vi "例4-7.vi"() -> ()   [LabVIEW 2019]
panel:
  out "所用时间9ms)":dbl
  out "执行次数":dbl
  in  "给定数据":dbl=50.0
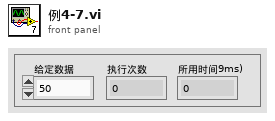
[diagram p1: front panel]
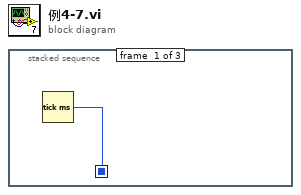
[diagram p0: block diagram]
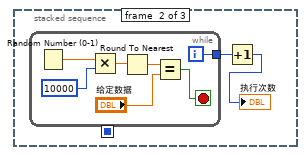
[diagram p2: hidden frame]
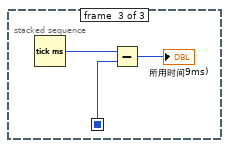
[diagram p3: hidden frame]
diagram:
  n1 = stacked-sequence {
    seq-local: [w1 _ _] -> [_ _ w12]
    frame #0 {
      n2 = Tick Count (ms)() -> (millisecond timer value=w1:u32)
    }
    frame #1 {
      n3 = while {
        tunnel: [w4] -> w3
        i -> [w4]
        stop <- w5 stop-if-true
        n4 = Random Number (0-1)() -> (number: 0 to 1=w9:dbl)
        n5 = Multiply(x=w9, y=10000) -> (x*y=w8:dbl)
        n6 = Round To Nearest(number=w8) -> (nearest integer value=w7:dbl)
        n7 = Equal?(x=w7, y="给定数据") -> (x = y?=w5:bool)
      }
      n8 = Increment(x=w3) -> (x+1=→"执行次数":i32)
    }
    frame #2 {
      n9 = Tick Count (ms)() -> (millisecond timer value=w13:u32)
      n10 = Subtract(x=w13, y=w12) -> (x-y=→"所用时间9ms)":u32)
    }
  }
